vi "Close Frame.vi"(8 "error in (no error)":errorcluster, 9 "timeout ms (5000)":i32=5000, 11 "WebSockets in":refnum<class "WebSocket.lvclass">) -> (0 "error out":errorcluster, 3 "WebSockets out":refnum<class "WebSocket.lvclass">)   [LabVIEW 2021, in "WebSockets.lvlib" / "WebSocket.lvclass"]
doc: "Sends a WebSocket close frame to the connection endpoint but does not close the underlying socket connection.\nWebSockets 2.0.1.40\nSam Sharp - MediaMongrels Ltd\nCopyright (c) 2019, MediaMongrels Ltd"
uses:
  WebSocket.lvclass
  Opcodes.ctl
  WebSocket.lvclass/WebSocket.ctl
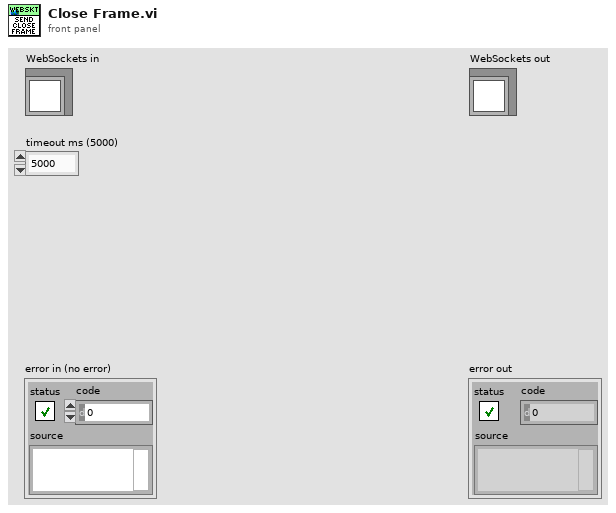
[diagram p1: front panel]
types:
  T1 = typedef "WebSockets.lvlib/WebSocket.lvclass/Opcodes.ctl" = u8
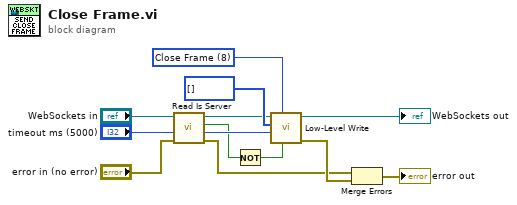
[diagram p0: block diagram]
diagram:
  w9 = T1 8 items=["Cont. Frame"=0, "Text"=1, "Binary"=2, "Close Frame"=8, "Ping"=9, "Pong"=10] ("Opcode (Text)")
  n1 = call-dynamic "Read Is Server.vi"("error in (no error)"="error in (no error)", "WebSocket in"="WebSockets in") -> ("error out"=w4:errorcluster, "Is Server?"=w3:bool, "WebSocket out"=w2:refnum<class "WebSocket.lvclass">)  [unwired: 7 in]
  n2 = Not(x=w3) -> (.not. x?=w6:bool)
  n3 = call "Low-Level Write.vi"("Mask payload?"=w6, "Opcode (Text)"=w9, "timeout ms (5000)"="timeout ms (5000)", "Data"=u8[] [], "WebSockets in"=w2) -> ("error out"=w12:errorcluster, "WebSockets out"=→"WebSockets out":refnum<class "WebSocket.lvclass">)  [unwired: 5 in]
  n4 = Merge Errors(w4, w12) -> (→"error out":errorcluster)
